vi "getParameters.vi"(11 "MoveHardpointActuatorsCommand in":refnum<class "MoveHardpointActuatorsCommand.lvclass">) -> (2 "Parameters":T1, 3 "MoveHardpointActuatorsCommand out":refnum<class "MoveHardpointActuatorsCommand.lvclass">)   [LabVIEW 2016, in "MoveHardpointActuatorsCommand.lvclass"]
uses:
  MoveHardpointActuatorsCommand.lvclass
  DataTypes/Topics/CommandMoveHardpointActuators.ctl
  DataTypes/Topics/Parts/CommandId.ctl
  MoveHardpointActuatorsCommand.lvclass/MoveHardpointActuatorsCommand.ctl
  DataTypes/Topics/M1M3SupportTopics.lvlib
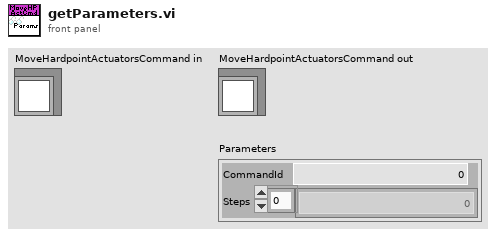
[diagram p1: front panel]
types:
  T1 = typedef "M1M3SupportTopics.lvlib/CommandMoveHardpointActuators.ctl" = cluster{"CommandId":T2, "Steps":i16[]}
  T2 = typedef "M1M3SupportTopics.lvlib/CommandId.ctl" = i32
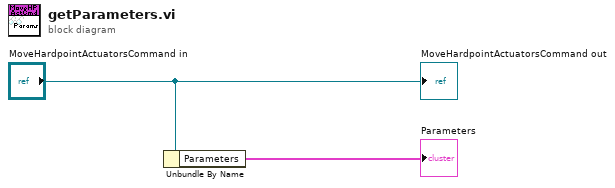
[diagram p0: block diagram]
diagram:
  n1 = Unbundle By Name("MoveHardpointActuatorsCommand in") -> ("Parameters"=→"Parameters":T1)
  "MoveHardpointActuatorsCommand out" <- "MoveHardpointActuatorsCommand in"
